vi "Create New Property Container.vi"(8 "error in (no error)":errorcluster, 11 "Engine in":refnum<class "Engine.lvclass">) -> (0 "error out":errorcluster, 2 "PropertyObject":T1, 3 "Engine out":refnum<class "Engine.lvclass">)   [LabVIEW 2020, in "TSS.lvlib" / "Engine.lvclass"]
uses:
  Engine.lvclass
  VariableContainer/Typedefs/Session Handle.ctl
  VariableContainer/VariableContainer.lvclass
  Engine.lvclass/Engine.ctl
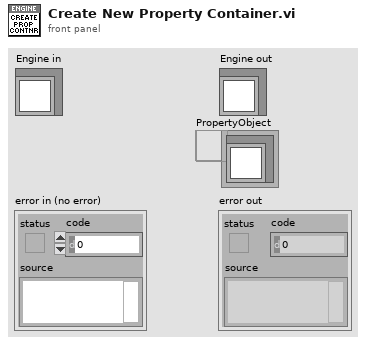
[diagram p1: front panel]
types:
  T1 = typedef "TSS.lvlib/VariableContainer.lvclass/Session Handle.ctl" = refnum<data-value>
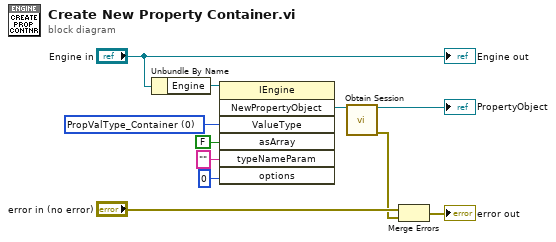
[diagram p0: block diagram]
diagram:
  w9 = 0 items=["PropValType_Container", "PropValType_String", "PropValType_Boolean", "PropValType_Number", "PropValType_NamedType", "PropValType_Reference", "PropValType_Array", "PropValType_Enum"] ("ValueType")
  n1 = Unbundle By Name("Engine in") -> ("Engine"=w10:refnum<k7>)
  n2 = invoke class="IEngine" method="NewPropertyObject"(reference=w10, "ValueType"=w9, "asArray"=FALSE, "typeNameParam"="", "options"=0) -> ("NewPropertyObject"=w8:refnum<k7>)  [unwired: 2 in, 6 out]
  n3 = call "Obtain Session.vi"("PropertyObject"=w8) -> ("Session Handle"=→"PropertyObject":T1, "error out"=w2:errorcluster)  [unwired: 13 in]
  n4 = Merge Errors("error in (no error)", w2) -> (→"error out":errorcluster)
  "Engine out" <- "Engine in"
